vi "Triekselfy.vi"(6 "Variant in":variant, 7 "Shift Pressed?":bool, 8 "error in":errorcluster, 10 "QD Combo Box Ref":refnum<vi>, 11 "QD Launch VI Ref":refnum<vi>) -> (0 "error out":errorcluster, 4 "Variant out":variant)   [LabVIEW 2021]
doc: "Nattification is the process by which a VI is modified to have the most sensible aesthetics and user-configurable options applied. This means non-terminal view on icons, left-justified subdiagram labels, autogrow disabled on all structures, etc.\n\nDefault Shortcut - [N]"
uses:
  <vilib>/Utility/traverseref.llb/TRef TravTarget.ctl
  <vilib>/Utility/Data Type/Type Definitions/Data Type.ctl
  <vilib>/Utility/traverseref.llb/VI Scripting - Traverse.lvlib
  <vilib>/Utility/Data Type/NI_Data Type.lvlib
panel:
  in  "Undo Name":string="Nattification"
  # "Many thanks to the Nattify quickdrop!"
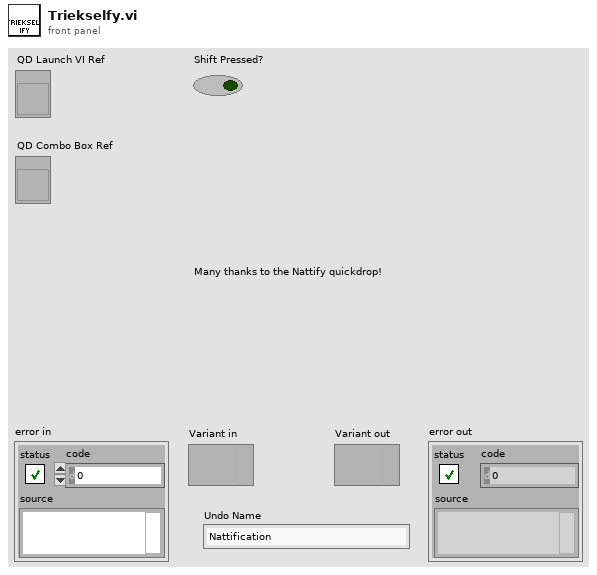
[diagram p1: front panel]
types:
  T1 = typedef "TRef TravTarget.ctl" = enum16{"FP", "BD", "Other"}
  T2 = typedef "NI_Data Type.lvlib/Data Type.ctl" = enum8{"Invalid Type", "Void", "I8", "I16", "I32", "I64", "U8", "U16", "U32", "U64", "Single Float", "Double Float", "Extended Float", "Single Complex", "Double Complex", "Extended Complex", "Enum U8", "Enum U16", "Enum U32", "Enum U64", "Single Float With Unit", "Double Float With Unit", "Extended Float With Unit", "Single Complex with Unit", "Double Complex with Unit", "Extended Complex with Unit", "Boolean", "String", "Path", "Picture", "Tag", "Array", "Cluster", "Variant", "LV Variant", "Waveform", "Timestamp", "Digital Waveform", "Digital Data", "ExpressData", "Refnum", "External Data", "VI", "Poly VI", "LabVIEW Class Instance", "Fixed Point", "Set Collection", "Map Collection"}
  T3 = enum16{"Auto Error Handling", "Autogrow", "Front Panel Color", "Icon View", "Move Error Wires Back", "Remove (no error)", "Subdiagram Label Justify", "Terminal Labels on Side", "Terminal Labels Transparent", "Color BD", "Arrange BD", "Separate compiled code from source file", "Arrange FP", "CamelCasing"}
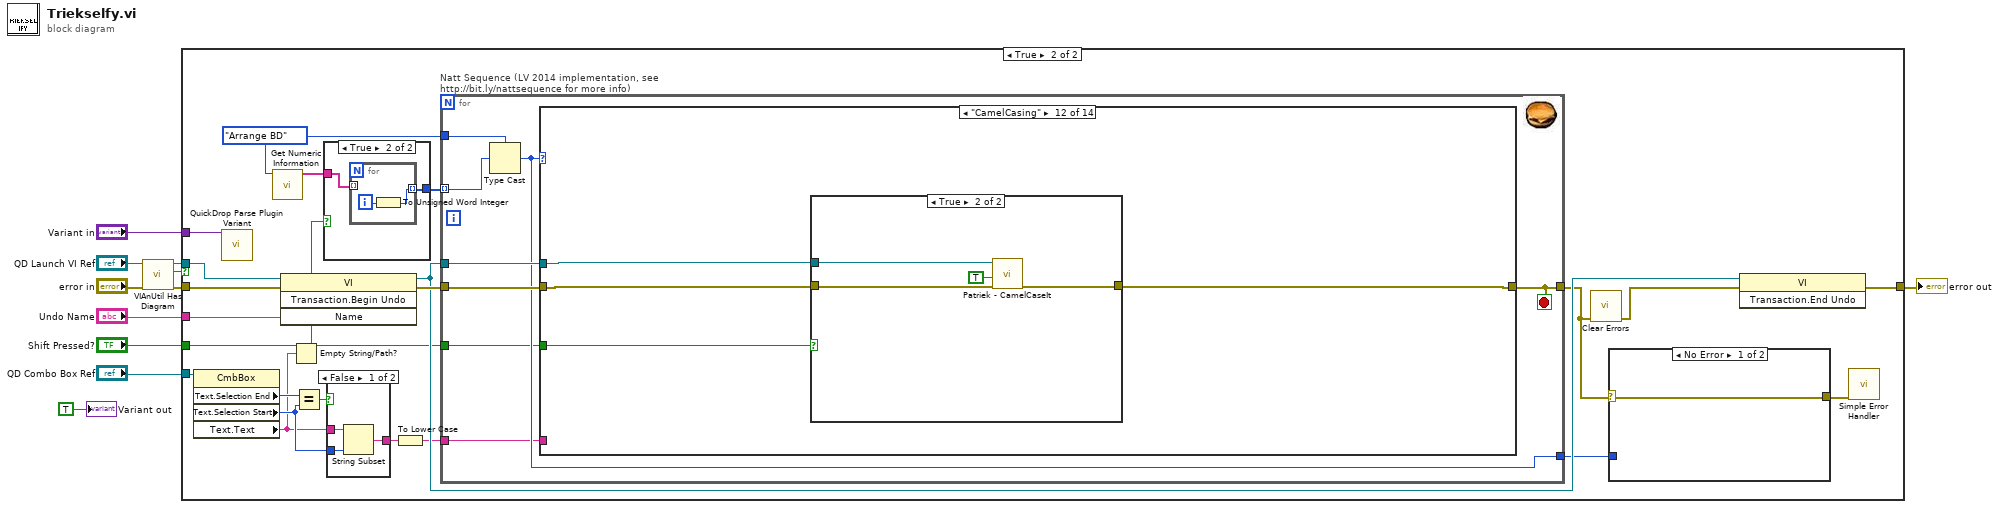
[diagram p0: block diagram]
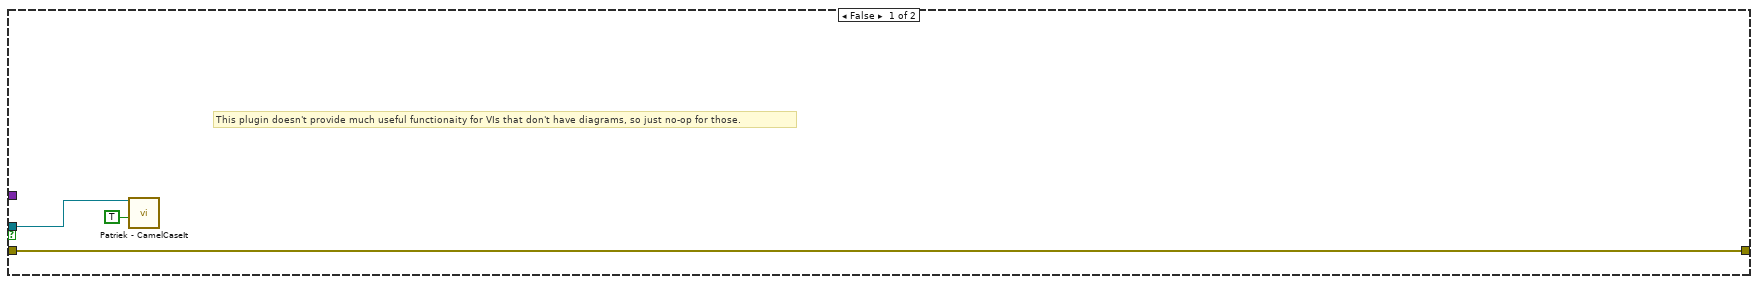
[diagram p2: hidden frame]
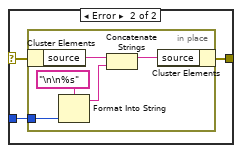
[diagram p3: hidden frame]
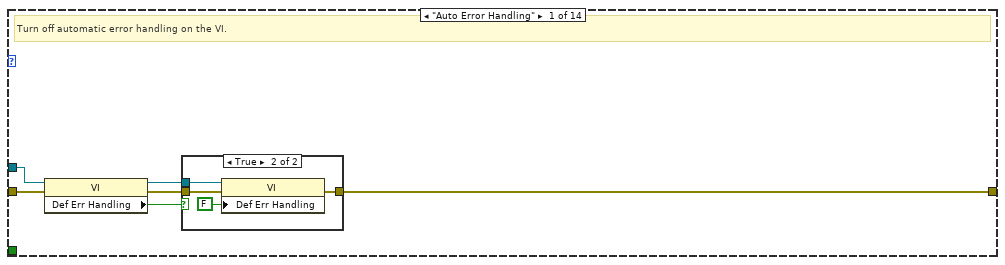
[diagram p4: hidden frame]
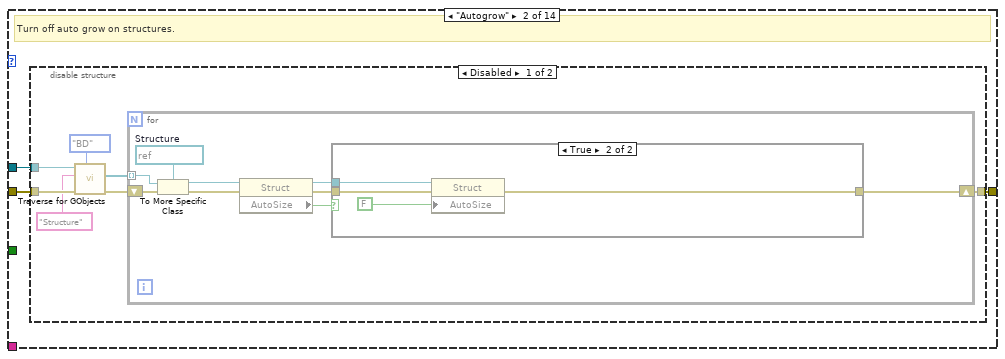
[diagram p6: hidden frame]
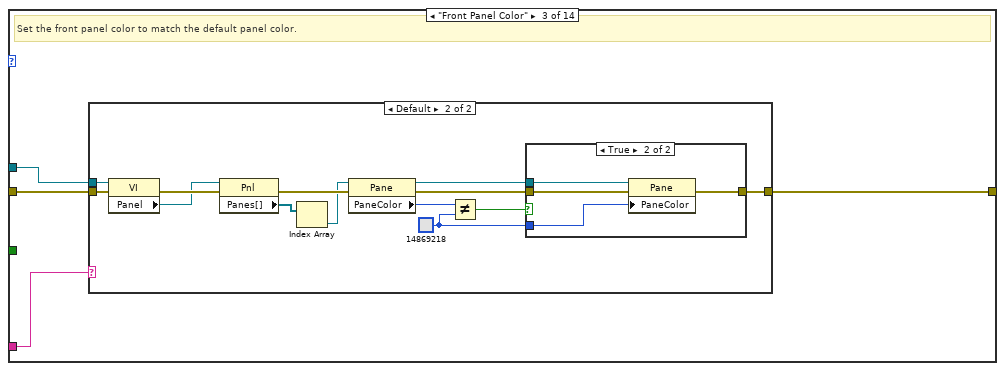
[diagram p9: hidden frame]
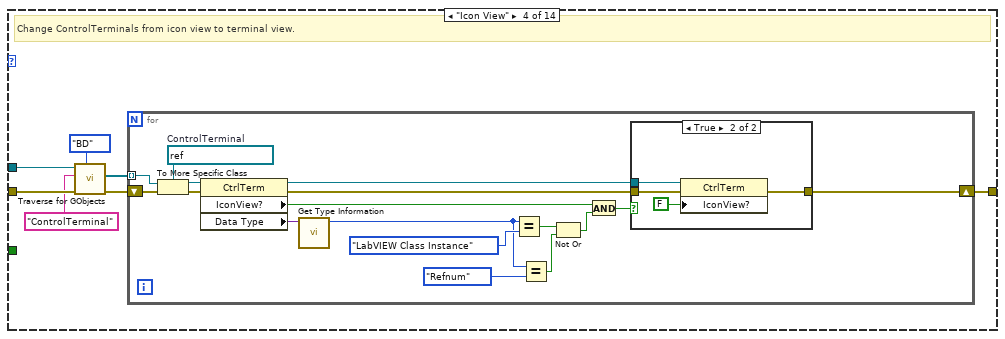
[diagram p12: hidden frame]
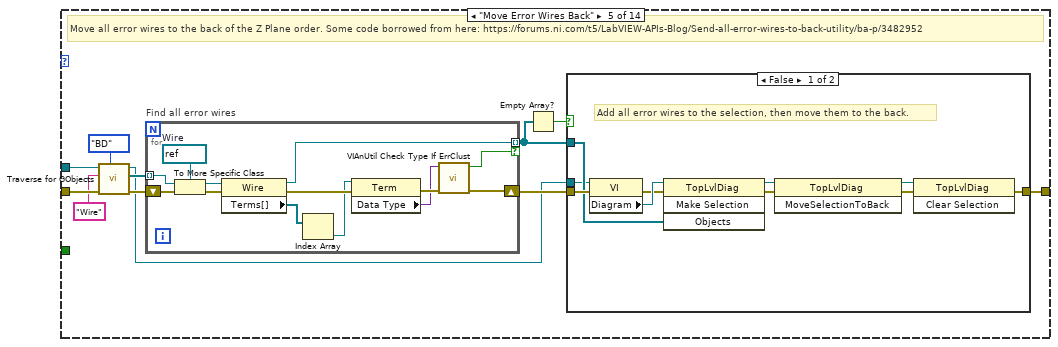
[diagram p14: hidden frame]
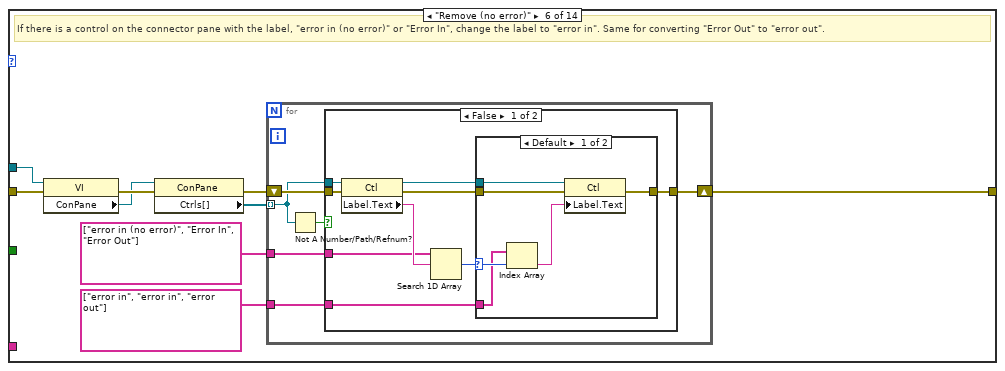
[diagram p16: hidden frame]
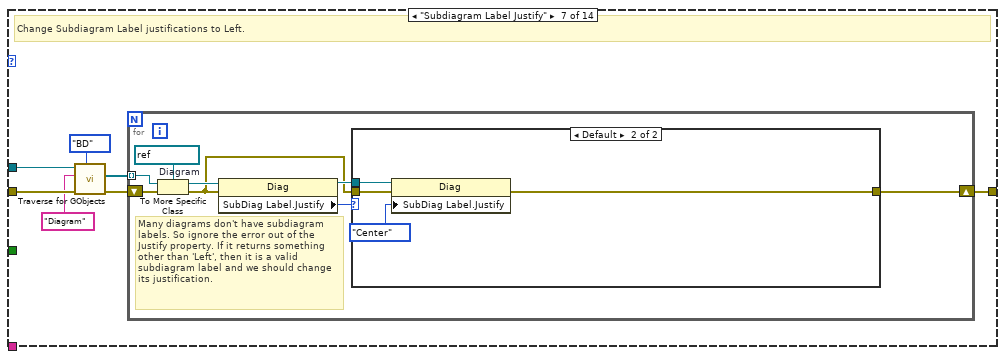
[diagram p19: hidden frame]
diagram:
  n1 = call <vilib>:"VIAnUtil Has Diagram.vi"("error in (no error)"="error in", "VI in"="QD Launch VI Ref") -> ("error out"=w6:errorcluster, "Has Diag?"=w3:bool, "VI out"=w4:refnum<vi>)  [unwired: 4 in, 3 out]
  n2 = case shown="True" w3 {
    tunnel: [w14 w37] -> w11
    tunnel: "Variant in" -> [_ w36]
    tunnel: "Undo Name" -> [_ w35]
    tunnel: w6 -> [w14 w32]
    tunnel: w4 -> [w13 w31]
    tunnel: "QD Combo Box Ref" -> [_ w22]
    tunnel: "Shift Pressed?" -> [_ w15]
    frame False {
      # "This plugin doesn't provide much useful functionaity for VIs that don't have diagrams, so just no-op for those."
      n3 = call <resource>:"Patriek - CamelCaseIt.vi"("MakeCamel"=TRUE, "VI in"=w13) -> ()  [unwired: 9 in, 1 out]
    }
    frame True {
      w18 = T3."Arrange BD"
      n4 = property on="Property Node" class="CmbBox"(reference=w22) -> ("Text.Selection End"=w26:u32, "Text.Selection Start"=w24:u32, "Text.Text"=w20:string)  [unwired: 1 in, 2 out]
      n5 = call <vilib>:"QuickDrop Parse Plugin Variant.vi"("QDKS Variant in"=w36) -> ()  [unwired: 12 in, 3 out]
      n6 = call <vilib>:"Get Numeric Information.vi"("variant"=w18) -> ("enum names"=w16:string[])  [unwired: 7 in, 3 out]
      n7 = invoke class="VI" method="Transaction.Begin Undo"(reference=w31, error in=w32, "Name"=w35) -> (reference out=w33:refnum<vi>, error out=w34:errorcluster)  [unwired: 1 in, 2 out]
      n8 = Empty String/Path?(string/path=w20) -> (empty?=w19:bool)
      n9 = Equal?(x=w26, y=w24) -> (x = y?=w25:bool)
      n10 = case shown="True" w19 {
        tunnel: [w286 w288] -> w17
        tunnel: w16 -> [w285 w287]
        frame False {
          n11 = call <resource>:"Enum Choice Array.vi"("Enum Names in"=w285) -> ("Array x"=w286:u16[])  [unwired: 10 in]
        }
        frame True {
          n12 = for {
            tunnel: w287 -> [_] mode=indexing
            tunnel: [w289] -> w288 mode=indexing
            i -> [w290]
            n13 = To Unsigned Word Integer(number=w290) -> (unsigned 16bit integer=w289:u16)
          }
        }
      }
      n14 = case shown="False" w25 {
        tunnel: [w293 w294] -> w23
        tunnel: w24 -> [w292 _]
        tunnel: w20 -> [w291 w294]
        frame False {
          n15 = String Subset(string=w291, length (rest)=w292) -> (substring=w293:string)  [unwired: 1 out]
        }
        frame True {
        }
      }
      n16 = To Lower Case(string=w23) -> (all lower case string=w21:string)
      n17 = for "Natt Sequence (LV 2014 implementation, see http://bit.ly/nattsequence for more info)" {
        tunnel: w18 -> [w54]
        tunnel: w34 -> [w53]
        tunnel: [w52] -> w29
        tunnel: w33 -> [w51]
        tunnel: [w50] -> w27
        tunnel: w21 -> [w49]
        tunnel: w17 -> [w48] mode=indexing
        tunnel: w15 -> [w47]
        stop <- w52 stop-if-true
        n18 = Type Cast(type=w54, x=w48) -> (*(type *) &x=w50:T3)
        n19 = case shown="\"CamelCasing\"" w50 {
          tunnel: w53 -> [w60 w68 w93 w119 w152 w185 w215 w231 w233 w248 w257 w265 w273 w278]
          tunnel: [w55 w66 w91 w113 w143 w178 w209 w229 w232 w249 w256 w264 w272 w274] -> w52
          tunnel: w51 -> [w59 w67 w92 w118 w151 w184 w214 w230 w234 w246 w255 w263 w271 w279]
          tunnel: w49 -> [_ _ w90 _ _ _ _ _ _ w247 _ _ _ _]
          tunnel: w47 -> [_ _ _ _ _ _ _ _ _ _ w254 w262 _ _]
          frame "Auto Error Handling" {
            # "Turn off automatic error handling on the VI."
            n20 = property class="VI"(reference=w59, error in=w60) -> (reference out=w56:refnum<vi>, error out=w58:errorcluster, "Def Err Handling"=w57:bool)
            n21 = case shown="True" w57 {
              tunnel: w58 -> [w61 w64]
              tunnel: w56 -> [_ w65]
              tunnel: [w61 w62] -> w55
              frame False {
              }
              frame True {
                n22 = property class="VI"(reference=w65, error in=w64, "Def Err Handling"=FALSE ("Automatic Error Handling")) -> (error out=w62:errorcluster)  [unwired: 1 out]
              }
            }
          }
          frame "Autogrow" {
            # "Turn off auto grow on structures."
            n23 = disable-structure shown="Disabled" {
              disable-tunnel: w68 -> [w75 _]
              disable-tunnel: w67 -> [w74 _]
              disable-tunnel: [w69 _] -> w66
              frame Disabled {
                n24 = call <vilib>:"Traverse for GObjects.vi"("Traverse Target"=TRef_TravTarget."BD", "error in (no error)"=w75, "Class Name"="Structure", "VI Refnum"=w74) -> ("error out"=w71:errorcluster, "References"=w70:refnum<vi>[])  [unwired: 4 in, 2 out]
                n25 = for {
                  shift-right: [w79] -> w69
                  shift-left: w71 -> [w84]
                  tunnel: w70 -> [w83] mode=indexing
                  w82 = refnum<vi> refnum  # Structure
                  n26 = To More Specific Class(target class=w82, reference=w83, error in=w84) -> (specific class reference=w81:refnum<vi>, error out=w80:errorcluster)
                  n27 = property class="Struct"(reference=w81, error in=w80) -> (reference out=w77:refnum<vi>, error out=w78:errorcluster, "AutoSize"=w76:bool)
                  n28 = case shown="True" w76 {
                    tunnel: [w85 w88] -> w79
                    tunnel: w78 -> [w85 w89]
                    tunnel: w77 -> [_ w87]
                    frame False {
                    }
                    frame True {
                      n29 = property class="Struct"(reference=w87, error in=w89, "AutoSize"=FALSE ("Icon View?")) -> (error out=w88:errorcluster)  [unwired: 1 out]
                    }
                  }
                }
              }
              frame Enabled {
              }
            }
          }
          frame "Front Panel Color" {
            # "Set the front panel color to match the default panel color."
            n30 = case shown="Default" w90 {
              tunnel: w93 -> [w94 w107]
              tunnel: w92 -> [_ w106]
              tunnel: [w94 w95] -> w91
              frame "p" {
                # "Don't change panel color if 'p' was typed"
              }
              frame Default {
                w99 = u32 14869218
                n31 = property class="VI"(reference=w106, error in=w107) -> (error out=w105:errorcluster, "Panel"=w104:refnum<vi>)  [unwired: 1 out]
                n32 = property class="Pnl"(reference=w104, error in=w105) -> (error out=w102:errorcluster, "Panes[]"=w103:refnum<vi>[])  [unwired: 1 out]
                n33 = Index Array(array=w103) -> (element=w101:refnum<vi>)  [unwired: 1 in]
                n34 = property class="Pane"(reference=w101, error in=w102) -> (reference out=w98:refnum<vi>, error out=w97:errorcluster, "PaneColor"=w96:u32)
                n35 = Not Equal?(x=w96, y=w99) -> (x != y?=w100:bool)
                n36 = case shown="True" w100 {
                  tunnel: [w108 w111] -> w95
                  tunnel: w97 -> [w108 w112]
                  tunnel: w98 -> [_ w110]
                  tunnel: w99 -> [_ w109]
                  frame False {
                  }
                  frame True {
                    n37 = property class="Pane"(reference=w110, error in=w112, "PaneColor"=w109) -> (error out=w111:errorcluster)  [unwired: 1 out]
                  }
                }
              }
            }
          }
          frame "Icon View" {
            # "Change ControlTerminals from icon view to terminal view."
            n38 = call <vilib>:"Traverse for GObjects.vi"("Traverse Target"=TRef_TravTarget."BD", "error in (no error)"=w119, "Class Name"="ControlTerminal", "VI Refnum"=w118) -> ("error out"=w115:errorcluster, "References"=w114:refnum<vi>[])  [unwired: 4 in, 2 out]
            n39 = for {
              shift-right: [w132] -> w113
              shift-left: w115 -> [w136]
              tunnel: w114 -> [w128] mode=indexing
              w135 = refnum<vi> refnum  # ControlTerminal
              n40 = To More Specific Class(target class=w135, reference=w128, error in=w136) -> (specific class reference=w134:refnum<vi>, error out=w133:errorcluster)
              n41 = property class="CtrlTerm"(reference=w134, error in=w133) -> (reference out=w130:refnum<vi>, error out=w131:errorcluster, "IconView?"=w129:bool, "Data Type"=w127:variant)
              n42 = call <vilib>:"Get Type Information.vi"("variant"=w127) -> ("type"=w124:T2)  [unwired: 6 in, 4 out]
              n43 = Equal?(x=w124, y=Data_Type."LabVIEW Class Instance" ("Type")) -> (x = y?=w123:bool)
              n44 = Equal?(x=w124, y=Data_Type."Refnum" ("Type")) -> (x = y?=w122:bool)
              n45 = Not Or(1:w122, 2:w123) -> (0:w120:bool)
              n46 = And(x=w129, y=w120) -> (x .and. y?=w121:bool)
              n47 = case shown="True" w121 {
                tunnel: [w137 w140] -> w132
                tunnel: w131 -> [w137 w141]
                tunnel: w130 -> [_ w139]
                frame False {
                }
                frame True {
                  n48 = property class="CtrlTerm"(reference=w139, error in=w141, "IconView?"=FALSE ("Icon View?")) -> (error out=w140:errorcluster)  [unwired: 1 out]
                }
              }
            }
          }
          frame "Move Error Wires Back" {
            # "Move all error wires to the back of the Z Plane order. Some code borrowed from here: https://forums.ni.com/t5/LabVIEW-APIs-Blog/Send-all-error-wires-to-back-utility/ba-p/3482952"
            n49 = call <vilib>:"Traverse for GObjects.vi"("Traverse Target"=TRef_TravTarget."BD", "error in (no error)"=w152, "Class Name"="Wire", "VI Refnum"=w151) -> ("error out"=w148:errorcluster, "References"=w147:refnum<vi>[], "dup VI Refnum"=w142:refnum<vi>)  [unwired: 4 in, 1 out]
            n50 = for "Find all error wires" {
              tunnel: w147 -> [w174] mode=indexing
              shift-right: [w164] -> w145
              shift-left: w148 -> [w176]
              tunnel: [w166] -> w144 mode=indexing if=w165
              w172 = refnum<vi> refnum  # Wire
              n51 = To More Specific Class(target class=w172, reference=w174, error in=w176) -> (specific class reference=w173:refnum<vi>, error out=w175:errorcluster)
              n52 = property class="Wire"(reference=w173, error in=w175) -> (reference out=w166:refnum<vi>, error out=w170:errorcluster, "Terms[]"=w171:refnum<vi>[])
              n53 = Index Array(array=w171) -> (element=w169:refnum<vi>)  [unwired: 1 in]
              n54 = property class="Term"(reference=w169, error in=w170) -> (error out=w168:errorcluster, "Data Type"=w167:variant)  [unwired: 1 out]
              n55 = call <vilib>:"VIAnUtil Check Type If ErrClust.vi"("error in (no error)"=w168, "Data In"=w167) -> ("error out"=w164:errorcluster, "IsErrClust?"=w165:bool)  [unwired: 8 in]
            }
            n56 = Empty Array?(array=w144) -> (empty?=w146:bool)
            n57 = case shown="False" w146 {
              tunnel: w145 -> [w159 w163]
              tunnel: w144 -> [w156 _]
              tunnel: [w154 w163] -> w143
              tunnel: w142 -> [w155 _]
              frame False {
                # "Add all error wires to the selection, then move them to the back."
                n58 = property class="VI"(reference=w155, error in=w159) -> (error out=w158:errorcluster, "Diagram"=w160:refnum<vi>)  [unwired: 1 out]
                n59 = invoke class="TopLvlDiag" method="Make Selection"(reference=w160, error in=w158, "Objects"=w156) -> (reference out=w162:refnum<vi>, error out=w161:errorcluster)  [unwired: 1 in, 2 out]
                n60 = invoke class="TopLvlDiag" method="MoveSelectionToBack"(reference=w162, error in=w161) -> (reference out=w153:refnum<vi>, error out=w157:errorcluster)  [unwired: 1 in, 1 out]
                n61 = invoke class="TopLvlDiag" method="Clear Selection"(reference=w153, error in=w157) -> (error out=w154:errorcluster)  [unwired: 1 in, 2 out]
              }
              frame True {
                # "No error wires on the diagram."
              }
            }
          }
          frame "Remove (no error)" {
            # "If there is a control on the connector pane with the label, \"error in (no error)\" or \"Error In\", change the label to \"error in\". Same for converting \"Error Out\" to \"error out\"."
            n62 = property class="VI"(reference=w184, error in=w185) -> (error out=w183:errorcluster, "ConPane"=w182:refnum<vi>)  [unwired: 1 out]
            n63 = property class="ConPane"(reference=w182, error in=w183) -> (error out=w181:errorcluster, "Ctrls[]"=w180:refnum<vi>[])  [unwired: 1 out]
            n64 = for {
              shift-right: [w189] -> w178
              shift-left: w181 -> [w191]
              tunnel: w180 -> [w187] mode=indexing
              tunnel: string[] ["error in (no error)", "Error In", "Error Out"] -> [w190]
              tunnel: string[] ["error in", "error in", "error out"] -> [w188]
              n65 = Not A Number/Path/Refnum?(number/path/refnum=w187) -> (NaN/Path/Refnum?=w186:bool)
              n66 = case shown="False" w186 {
                tunnel: w191 -> [w200 w208]
                tunnel: w187 -> [w199 _]
                tunnel: w190 -> [w197 _]
                tunnel: [w194 w208] -> w189
                tunnel: w188 -> [w192 _]
                frame False {
                  n67 = property class="Ctl"(reference=w199, error in=w200) -> (reference out=w193:refnum<vi>, error out=w196:errorcluster, "Label.Text"=w198:string)
                  n68 = Search 1D Array(1D array=w197, element=w198) -> (index of element=w195:i32)  [unwired: 1 in]
                  n69 = case shown="Default" w195 {
                    selector: w195 -> [w203 _]
                    tunnel: w196 -> [w204 w207]
                    tunnel: [w205 w207] -> w194
                    tunnel: w193 -> [w206 _]
                    tunnel: w192 -> [w202 _]
                    frame Default {
                      n70 = Index Array(array=w202, index=w203) -> (element=w201:string)
                      n71 = property class="Ctl"(reference=w206, error in=w204, "Label.Text"=w201) -> (error out=w205:errorcluster)  [unwired: 1 out]
                    }
                    frame -1 {
                    }
                  }
                }
                frame True {
                  # "Empty spot on the conpane, ignore it."
                }
              }
            }
          }
          frame "Subdiagram Label Justify" {
            # "Change Subdiagram Label justifications to Left."
            n72 = call <vilib>:"Traverse for GObjects.vi"("Traverse Target"=TRef_TravTarget."BD", "error in (no error)"=w215, "Class Name"="Diagram", "VI Refnum"=w214) -> ("error out"=w211:errorcluster, "References"=w210:refnum<vi>[])  [unwired: 4 in, 2 out]
            n73 = for {
              shift-right: [w216] -> w209
              shift-left: w211 -> [w223]
              tunnel: w210 -> [w222] mode=indexing
              w221 = refnum<vi> refnum  # Diagram
              # "Many diagrams don't have subdiagram labels. So ignore the error out of the Justify property. If it returns something other than 'Left', then it is a valid subdiagram label and we should change its justification."
              n74 = To More Specific Class(target class=w221, reference=w222, error in=w223) -> (specific class reference=w220:refnum<vi>, error out=w217:errorcluster)
              n75 = property class="Diag"(reference=w220, error in=w217) -> (reference out=w218:refnum<vi>, "SubDiag Label.Justify"=w219:enum16{"Left", "Center", "Right"})  [unwired: 1 out]
              n76 = case shown="Default" w219 {
                tunnel: w218 -> [_ w228]
                tunnel: w217 -> [w224 w227]
                tunnel: [w224 w226] -> w216
                frame "Left" {
                }
                frame Default {
                  n77 = property class="Diag"(reference=w228, error in=w227, "SubDiag Label.Justify"=enum16{"Left", "Center", "Right"}."Center" ("Subdiagram Label.Justification")) -> (error out=w226:errorcluster)  [unwired: 1 out]
                }
              }
            }
          }
          frame "Terminal Labels on Side" {
            # "Move control and indicator terminal labels to the sides. Code borrowed from here: resource\\dialog\\QuickDrop\\plugins\\Move Labels.vi"
            n78 = call <resource>:"Patriek - Align Terminals.vi"("error in (no error)"=w231, "VI in"=w230) -> ("error out"=w229:errorcluster)  [unwired: 9 in]
          }
          frame "Terminal Labels Transparent" {
            # "Make all control terminal labels have transparent backgrounds."
            n79 = call <vilib>:"Traverse for GObjects.vi"("Traverse Target"=TRef_TravTarget."BD", "error in (no error)"=w233, "Class Name"="ControlTerminal", "VI Refnum"=w234) -> ("error out"=w236:errorcluster, "References"=w235:refnum<vi>[])  [unwired: 4 in, 2 out]
            n80 = for {
              shift-right: [w240] -> w232
              shift-left: w236 -> [w245]
              tunnel: w235 -> [w244] mode=indexing
              w239 = u32 16777216
              w243 = refnum<vi> refnum  # ControlTerminal
              n81 = To More Specific Class(target class=w243, reference=w244, error in=w245) -> (specific class reference=w242:refnum<vi>, error out=w241:errorcluster)
              n82 = property class="CtrlTerm"(reference=w242, error in=w241, "Label.BG Color"=w239, "Label.FG Color"=w239, "Label.BGColor"=w239) -> (error out=w240:errorcluster)  [unwired: 1 out]
            }
          }
          frame "Arrange FP" {
            # "Clean up front panel and position/resize it properly.  Do this action last since previous actions might move things around."
            n83 = case shown="Default" w247 {
              tunnel: [w250 w253] -> w249
              tunnel: w248 -> [w250 w252]
              tunnel: w246 -> [_ w251]
              frame "p" {
                # "don't arrange panel if 'p' was typed"
              }
              frame Default {
                n84 = call <resource>:"Nattify - Arrange FP.vi"("VI in"=w251, "error in"=w252) -> ("error out"=w253:errorcluster)  [unwired: 12 in, 1 out]
              }
            }
          }
          frame "Color BD" {
            n85 = case shown="True" w254 {
              tunnel: w257 -> [w258 w261]
              tunnel: [w258 w260] -> w256
              tunnel: w255 -> [_ w259]
              frame False {
              }
              frame True {
                n86 = call <resource>:"Patriek - Color Block Diagram.vi"("error in (no error)"=w261, "VI in"=w259) -> ("error out"=w260:errorcluster)  [unwired: 9 in]
              }
            }
          }
          frame "CamelCasing" {
            n87 = case shown="True" w262 {
              tunnel: w265 -> [w266 w270]
              tunnel: [w266 w269] -> w264
              tunnel: w263 -> [_ w268]
              frame False {
              }
              frame True {
                n88 = call <resource>:"Patriek - CamelCaseIt.vi"("error in (no error)"=w270, "MakeCamel"=TRUE, "VI in"=w268) -> ("error out"=w269:errorcluster)  [unwired: 8 in]
              }
            }
          }
          frame "Arrange BD" {
            # "Position/resize block diagram window. Do this action last since previous actions might move things around."
            n89 = call <resource>:"Nattify - Arrange BD.vi"("VI in"=w271, "error in"=w273) -> ("error out"=w272:errorcluster)  [unwired: 13 in]
          }
          frame "Separate compiled code from source file" {
            n90 = property class="VI"(reference=w279, error in=w278) -> (reference out=w276:refnum<vi>, error out=w275:errorcluster, "ContainstCompiledCode"=w277:bool)
            n91 = case shown="True" w277 {
              tunnel: w276 -> [_ w284]
              tunnel: w275 -> [w280 w283]
              tunnel: [w280 w281] -> w274
              frame False {
              }
              frame True {
                w282 = FALSE  # Contains Compiled Code
                n92 = property class="VI"(reference=w284, error in=w283, "ContainstCompiledCode"=w282) -> (error out=w281:errorcluster)  [unwired: 1 out]
              }
            }
          }
        }
      }
      n93 = call <vilib>:"Clear Errors.vi"("error in (no error)"=w29) -> ("error out"=w30:errorcluster)  [unwired: 5 in, 1 out]
      n94 = case shown="No Error" w29 {
        selector: w29 -> [w38 w41]
        tunnel: [w38 w40] -> w28
        tunnel: w27 -> [_ w39]
        frame No Error {
        }
        frame Error {
          n95 = in-place {
            in-place-border: w39 -> [w42]
            n96 = in-place-cluster #1(w41) -> ("source"=w46:string)
            n97 = Format Into String(format string="\n\n%s", w42) -> (resulting string=w44:string)  [unwired: 2 in, 1 out]
            n98 = Concatenate Strings(w46, w44) -> (w45:string)
            n99 = in-place-cluster #1("source"=w45) -> (w40:errorcluster)
          }
        }
      }
      n100 = invoke class="VI" method="Transaction.End Undo"(reference=w33, error in=w30) -> (error out=w37:errorcluster)  [unwired: 1 in, 2 out]
      n101 = call <vilib>:"Simple Error Handler.vi"("error in (no error)"=w28) -> ()  [unwired: 4 in, 5 out]
    }
  }
  "error out" <- w11
  "Variant out" <- TRUE
